vi "SubVI_DriveStraightning_Teleop.vi"(9 "Y Input":dbl, 10 "X Input":dbl) -> (1 "Y Output":dbl, 2 "X Output":dbl)   [LabVIEW 2017]
uses:
  <vilib>/Rock Robotics/WPI/ThirdParty/Sensors/navX/_TypeDefs/FRIC_navX_DeviceNumbersTypeDef.ctl
panel:
  in  "D Gain":dbl
  in  "P Gain":dbl
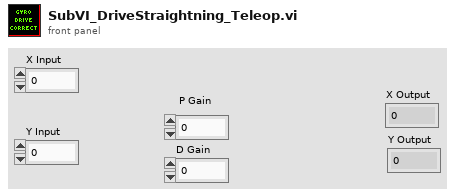
[diagram p1: front panel]
types:
  T1 = typedef "FRIC_navX_DeviceNumbersTypeDef.ctl" = enum16{"Dev0", "Dev1", "Dev2", "Dev3"}
  T2 = cluster{"Yaw":dbl, "Roll":dbl, "Pitch":dbl, "Heading":dbl, "Fused Heading":dbl}
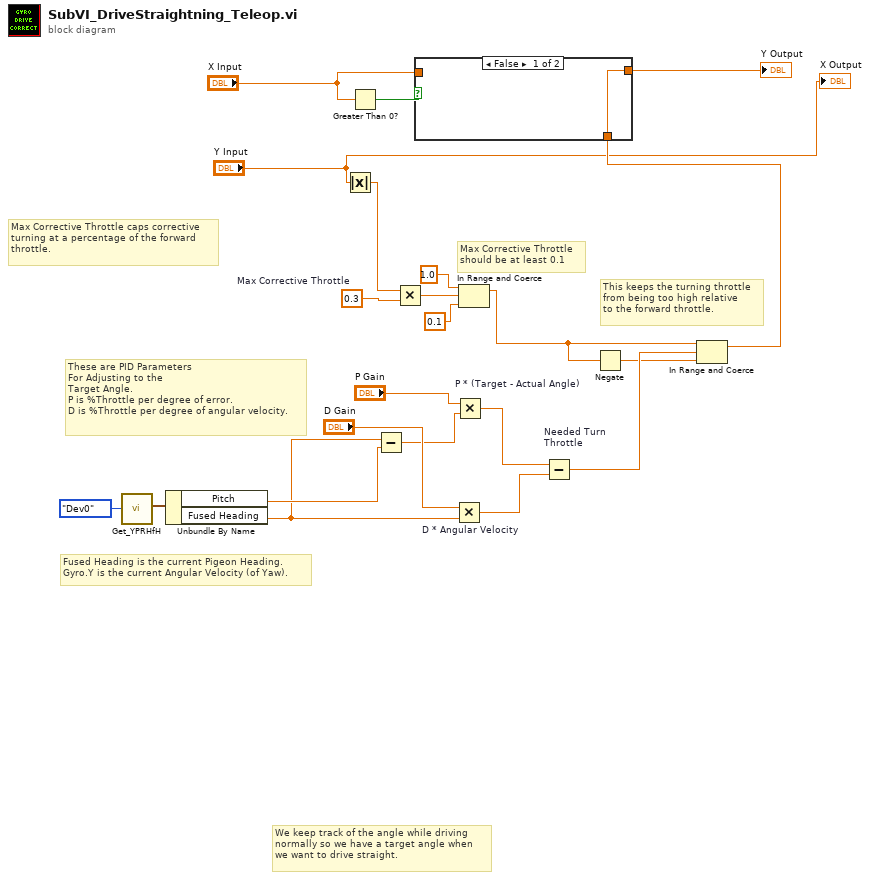
[diagram p0: block diagram]
diagram:
  w22 = 0.3  # Max Corrective Throttle
  # "This keeps the turning throttle\nfrom being too high relative\nto the forward throttle."
  # "Max Corrective Throttle\nshould be at least 0.1"
  # "Fused Heading is the current Pigeon Heading.\nGyro.Y is the current Angular Velocity (of Yaw)."
  # "Max Corrective Throttle caps corrective\nturning at a percentage of the forward\nthrottle."
  # "We keep track of the angle while driving\nnormally so we have a target angle when\nwe want to drive straight."
  # "These are PID Parameters\nFor Adjusting to the\nTarget Angle.\nP is %Throttle per degree of error.\nD is %Throttle per degree of angular velocity."
  n1 = call <vilib>:"Get_YPRHfH.vi"("Device Number"=FRIC_navX_DeviceNumbersTypeDef."Dev0") -> ("YRPHfH"=w18:T2)  [unwired: 10 in]
  n2 = Unbundle By Name(w18) -> ("Pitch"=w17:dbl, "Fused Heading"=w4:dbl)
  n3 = Absolute Value(x="Y Input") -> (abs(x)=w13:dbl)
  n4 = Greater Than 0?(x="X Input") -> (x > 0?=w6:bool)
  n5 = Subtract(x=w4, y=w17) -> (x-y=w16:dbl)
  n6 = Multiply ("P * (Target - Actual Angle)")(x=w13, y=w22) -> (x*y=w10:dbl)
  n7 = Multiply "D * Angular Velocity"(x="D Gain", y=w4) -> (x*y=w14:dbl)
  n8 = Multiply "P * (Target - Actual Angle)"(x="P Gain", y=w16) -> (x*y=w15:dbl)
  n9 = In Range and Coerce(upper limit=1.0, x=w10, lower limit=0.1) -> (coerced(x)=w8:dbl)  [unwired: 1 out]
  n10 = Subtract "Needed Turn \nThrottle"(x=w15, y=w14) -> (x-y=w9:dbl)
  n11 = Negate(x=w8) -> (-x=w7:dbl)
  n12 = In Range and Coerce(upper limit=w8, x=w9, lower limit=w7) -> (coerced(x)=w5:dbl)  [unwired: 1 out]
  n13 = case shown="False" w6 {
    tunnel: [w23 w24] -> w3
    tunnel: w5 -> [w23 _]
    tunnel: "X Input" -> [_ w24]
    frame False {
    }
    frame True {
    }
  }
  "Y Output" <- w3
  "X Output" <- "Y Input"
